vi "BernoulliNB.vi"(8 "error in":errorcluster) -> (0 "error out":errorcluster, 3 "out":refnum<class "BernoulliNB.lvclass">)   [LabVIEW 2020]
doc: "Naive Bayes classifier for multivariate Bernoulli models.\n\n Like MultinomialNB, this classifier is suitable for discrete data. The\n difference is that while MultinomialNB works with occurrence counts,\n BernoulliNB is designed for binary/boolean features.\n\n Read more in the :ref:`User Guide <bernoulli_naive_bayes>`.\n\n Parameters\n ----------\n alpha : float, default=1.0\n Additive (Laplace/Lidstone) smoothing parameter\n (0 for no smoothing).\n\n binarize : float or None, default=0.0\n Threshold for binarizing (mapping to booleans) of sample features.\n If None, input is presumed to already consist of binary vectors.\n\n fit_prior : bool, default=True\n Whether to learn class prior probabilities or not.\n If false, a uniform prior will be used.\n\n class_prior : array-like of shape (n_classes,), default=None\n Prior probabilities of the classes. If specified the priors are not\n adjusted according to the data.\n\n Attributes\n ----------\n class_count_ : ndarray of shape (n_classes)\n Number of samples encountered for each class during fitting. This\n value is weighted by the sample weight when provided.\n\n class_log_prior_ : ndarray of shape (n_classes)\n Log probability of each class (smoothed).\n\n classes_ : ndarray of shape (n_classes,)\n Class labels known to the classifier\n\n coef_ : ndarray of shape (n_classes, n_features)\n Mirrors ``feature_log_prob_`` for interpreting `BernoulliNB`\n as a linear model.\n\n feature_count_ : ndarray of shape (n_classes, n_features)\n Number of samples encountered for each (class, feature)\n during fitting. This value is weighted by the sample weight when\n provided.\n\n feature_log_prob_ : ndarray of shape (n_classes, n_features)\n Empirical log probability of features given a class, P(x_i|y).\n\n intercept_ : ndarray of shape (n_classes,)\n Mirrors ``class_log_prior_`` for interpreting `BernoulliNB`\n as a linear model.\n\n n_features_ : int\n Number of features of each sample.\n\n \nAvailable methods:\nFit\nPartial Fit\nPredict\nPredict Log Proba\nPredict Proba\nScore\nGet Attributes\nGet Params\nSet Params"
uses:
  BernoulliNB.lvclass
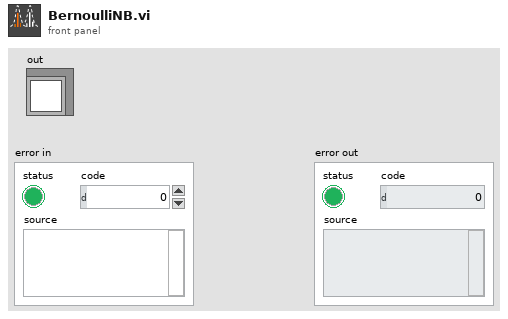
[diagram p1: front panel]
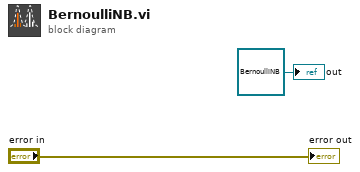
[diagram p0: block diagram]
diagram:
  "out" <- refnum<class "BernoulliNB.lvclass"> refnum ("model")
  "error out" <- "error in"
